vi "Data Parameters FG.vi"(7 "Action":T1, 8 "error in (no error)":errorcluster, 10 "Data Parameters":T3={"Data Type"=enum."Single Channel", "Channel Type"=enum."Format", "Format String"="%.3g", "Expected String"="", "Type"=enum."SGL", "List"=[], "Delimiter"=","}, 11 "Item Ref in":T2 format="%.0x") -> (0 "error out":errorcluster, 2 "Data Parameters":T3={"Data Type"=enum."Single Channel", "Channel Type"=enum."Format", "Format String"="%.3g", "Expected String"="", "Type"=enum."SGL", "List"=[], "Delimiter"=","}, 3 "Item Ref out":T2 format="%.0x")   [LabVIEW 2015, in "Instrument Addon Shared.lvlib"]
uses:
  Instrument Addon Shared.lvlib
  Types/Data Parameters.ctl
  Types/Protocol Data Type.ctl
  Types/Data Channel Type.ctl
  Types/Type Cast Type.ctl
  <vilib>/NI Veristand/Custom Device API/Custom Device Item Ref.ctl
  Types/FG Control.ctl
  <vilib>/NI Veristand/Custom Device API/Set Item Property (String).vi
  <vilib>/NI Veristand/Custom Device API/Set Item Property (String Array).vi
  <vilib>/NI Veristand/Custom Device API/Set Item Property (U32).vi
  <vilib>/NI Veristand/Custom Device API/Get Item Property (String).vi
  <vilib>/NI Veristand/Custom Device API/Get Item Property (String Array).vi
  <vilib>/NI Veristand/Custom Device API/Get Item Property (U32).vi
  Constants.vi
  <vilib>/NI VeriStand/Custom Device API/Custom Device API.lvlib
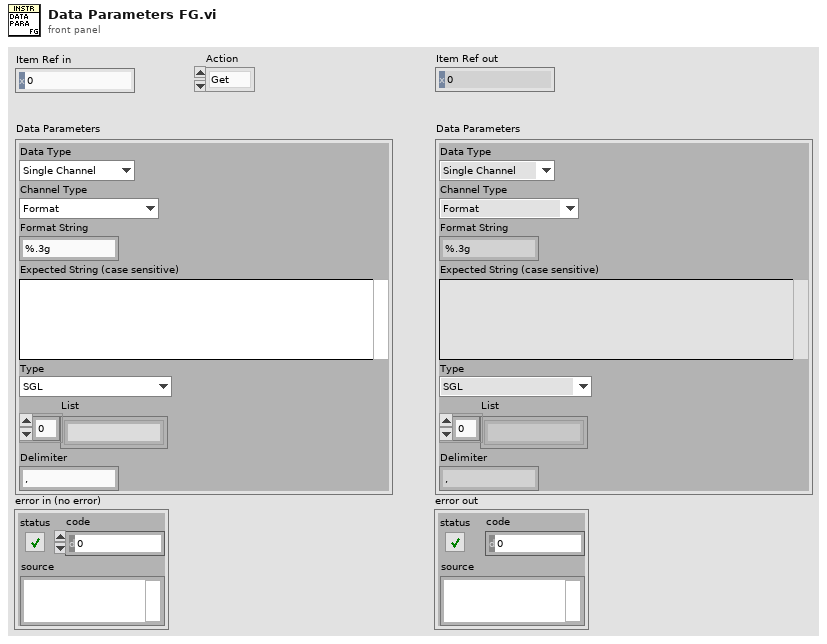
[diagram p1: front panel]
types:
  T1 = typedef "Instrument Addon Shared.lvlib/FG Control.ctl" = enum16{"Get", "Set"}
  T2 = typedef "Custom Device API.lvlib/Custom Device Item Ref.ctl" = u64
  T3 = typedef "Instrument Addon Shared.lvlib/Data Parameters.ctl" = cluster{"Data Type":T4, "Channel Type":T5, "Format String":string, "Expected String":string, "Type":T6, "List":string[], "Delimiter":string}
  T4 = typedef "Instrument Addon Shared.lvlib/Protocol Data Type.ctl" = enum16{"Single Channel", "Array"}
  T5 = typedef "Instrument Addon Shared.lvlib/Data Channel Type.ctl" = enum16{"Format", "Comparison", "Type Cast", "Enumerated List"}
  T6 = typedef "Instrument Addon Shared.lvlib/Type Cast Type.ctl" = enum16{"DBL", "SGL", "U64", "U32", "U16", "U8", "I64", "I32", "I16", "I8"}
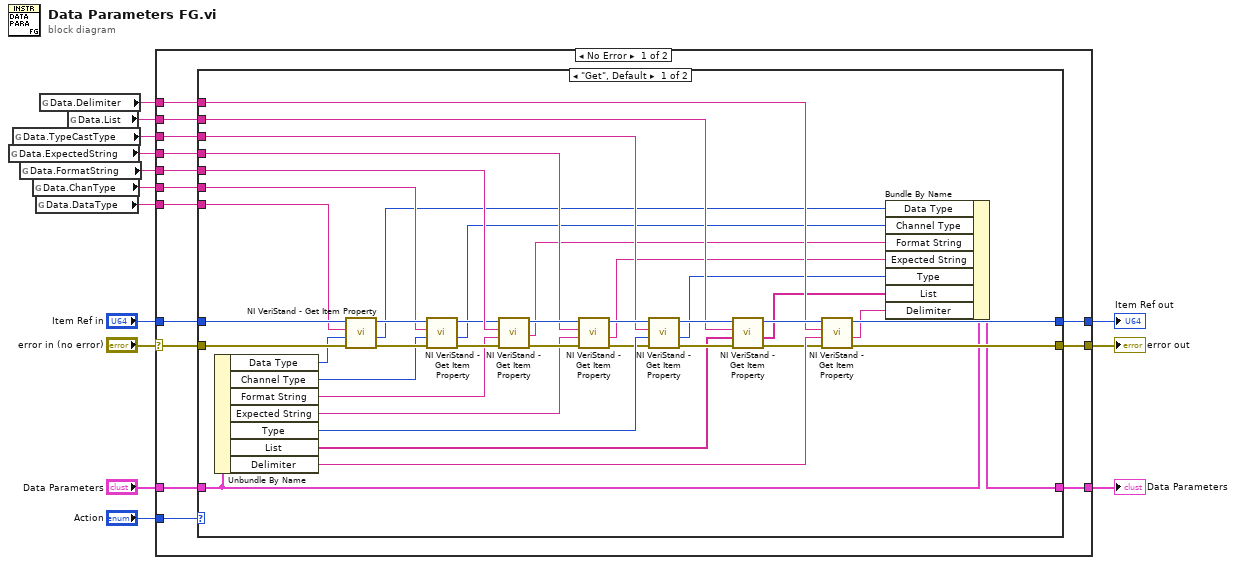
[diagram p0: block diagram]
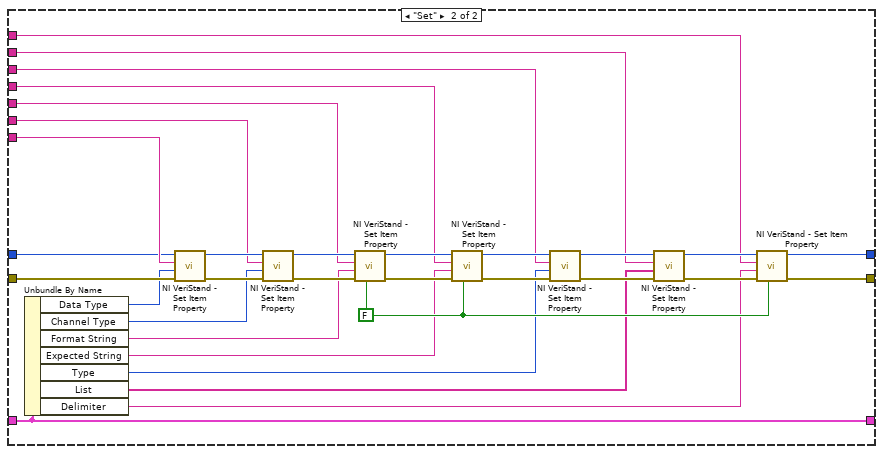
[diagram p2: hidden frame]
diagram:
  n1 = global read "Constants.vi" "Data.ExpectedString"() -> (w4:string)
  n2 = global read "Constants.vi" "Data.TypeCastType"() -> (w3:string)
  n3 = global read "Constants.vi" "Data.FormatString"() -> (w5:string)
  n4 = global read "Constants.vi" "Data.ChanType"() -> (w6:string)
  n5 = global read "Constants.vi" "Data.DataType"() -> (w8:string)
  n6 = global read "Constants.vi" "Data.Delimiter"() -> (w1:string)
  n7 = global read "Constants.vi" "Data.List"() -> (w2:string)
  n8 = case shown="No Error" "error in (no error)" {
    selector: "error in (no error)" -> [w23 w102]
    tunnel: w8 -> [w28 _]
    tunnel: [w27 w100] -> w12
    tunnel: "Item Ref in" -> [w26 w100]
    tunnel: "Data Parameters" -> [w25 w101]
    tunnel: [w24 w102] -> w11
    tunnel: [w22 w101] -> w7
    tunnel: "Action" -> [w21 _]
    tunnel: w6 -> [w20 _]
    tunnel: w5 -> [w19 _]
    tunnel: w4 -> [w18 _]
    tunnel: w3 -> [w17 _]
    tunnel: w2 -> [w16 _]
    tunnel: w1 -> [w15 _]
    frame No Error {
      n9 = case shown="\"Get\", Default" w21 {
        tunnel: w28 -> [w65 w99]
        tunnel: [w42 w82] -> w27
        tunnel: w26 -> [w66 w98]
        tunnel: w25 -> [w37 w96]
        tunnel: [w46 w83] -> w24
        tunnel: w23 -> [w67 w97]
        tunnel: [w36 w96] -> w22
        tunnel: w20 -> [w60 w73]
        tunnel: w19 -> [w59 w72]
        tunnel: w18 -> [w41 w71]
        tunnel: w17 -> [w40 w70]
        tunnel: w16 -> [w39 w69]
        tunnel: w15 -> [w38 w68]
        frame "Get", Default {
          n10 = Unbundle By Name(w37) -> ("Data Type"=w64:T4, "Channel Type"=w61:T5, "Format String"=w56:string, "Expected String"=w53:string, "Type"=w52:T6, "List"=w48:string[], "Delimiter"=w47:string)
          n11 = call-poly <vilib>:"NI VeriStand - Get Item Property.vi"("error in (no error)"=w67, "Default Value"=w64, "Property Name"=w65, "Item Ref in"=w66) -> ("error out"=w62:errorcluster, "Value"=w29:u32, "Item Ref out"=w63:T2)  [unwired: 4 in, 1 out]
          n12 = call-poly <vilib>:"NI VeriStand - Get Item Property.vi"("error in (no error)"=w62, "Default Value"=w61, "Property Name"=w60, "Item Ref in"=w63) -> ("error out"=w57:errorcluster, "Value"=w30:u32, "Item Ref out"=w58:T2)  [unwired: 4 in, 1 out]
          n13 = call-poly <vilib>:"NI VeriStand - Get Item Property.vi"("error in (no error)"=w57, "Default Value"=w56, "Property Name"=w59, "Item Ref in"=w58) -> ("error out"=w54:errorcluster, "Value"=w31:string, "Item Ref out"=w55:T2)  [unwired: 4 in, 1 out]
          n14 = call-poly <vilib>:"NI VeriStand - Get Item Property.vi"("error in (no error)"=w54, "Default Value"=w53, "Property Name"=w41, "Item Ref in"=w55) -> ("error out"=w51:errorcluster, "Value"=w32:string, "Item Ref out"=w50:T2)  [unwired: 4 in, 1 out]
          n15 = call-poly <vilib>:"NI VeriStand - Get Item Property.vi"("error in (no error)"=w51, "Default Value"=w52, "Property Name"=w40, "Item Ref in"=w50) -> ("error out"=w49:errorcluster, "Value"=w33:u32, "Item Ref out"=w44:T2)  [unwired: 4 in, 1 out]
          n16 = call-poly <vilib>:"NI VeriStand - Get Item Property.vi"("error in (no error)"=w49, "Default Value"=w48, "Property Name"=w39, "Item Ref in"=w44) -> ("error out"=w45:errorcluster, "Value"=w34:string[], "Item Ref out"=w43:T2)  [unwired: 4 in, 1 out]
          n17 = call-poly <vilib>:"NI VeriStand - Get Item Property.vi"("error in (no error)"=w45, "Default Value"=w47, "Property Name"=w38, "Item Ref in"=w43) -> ("error out"=w46:errorcluster, "Value"=w35:string, "Item Ref out"=w42:T2)  [unwired: 4 in, 1 out]
          n18 = Bundle By Name(cluster=w37, "Data Type"=w29, "Channel Type"=w30, "Format String"=w31, "Expected String"=w32, "Type"=w33, "List"=w34, "Delimiter"=w35) -> (w36:T3)
        }
        frame "Set" {
          w78 = FALSE ("Binary String (T)")
          n19 = Unbundle By Name(w96) -> ("Data Type"=w81:T4, "Channel Type"=w80:T5, "Format String"=w79:string, "Expected String"=w77:string, "Type"=w76:T6, "List"=w75:string[], "Delimiter"=w74:string)
          n20 = call-poly <vilib>:"NI VeriStand - Set Item Property.vi"("error in (no error)"=w97, "Value"=w81, "Property Name"=w99, "Item Ref in"=w98) -> ("error out"=w94:errorcluster, "Item Ref out"=w95:T2)  [unwired: 5 in, 1 out]
          n21 = call-poly <vilib>:"NI VeriStand - Set Item Property.vi"("error in (no error)"=w94, "Value"=w80, "Property Name"=w73, "Item Ref in"=w95) -> ("error out"=w92:errorcluster, "Item Ref out"=w93:T2)  [unwired: 5 in, 1 out]
          n22 = call-poly <vilib>:"NI VeriStand - Set Item Property.vi"("Binary String (T)"=w78, "error in (no error)"=w92, "Value"=w79, "Property Name"=w72, "Item Ref in"=w93) -> ("error out"=w90:errorcluster, "Item Ref out"=w91:T2)  [unwired: 4 in, 1 out]
          n23 = call-poly <vilib>:"NI VeriStand - Set Item Property.vi"("Binary String (T)"=w78, "error in (no error)"=w90, "Value"=w77, "Property Name"=w71, "Item Ref in"=w91) -> ("error out"=w88:errorcluster, "Item Ref out"=w89:T2)  [unwired: 4 in, 1 out]
          n24 = call-poly <vilib>:"NI VeriStand - Set Item Property.vi"("error in (no error)"=w88, "Value"=w76, "Property Name"=w70, "Item Ref in"=w89) -> ("error out"=w87:errorcluster, "Item Ref out"=w86:T2)  [unwired: 5 in, 1 out]
          n25 = call-poly <vilib>:"NI VeriStand - Set Item Property.vi"("error in (no error)"=w87, "Value"=w75, "Property Name"=w69, "Item Ref in"=w86) -> ("error out"=w85:errorcluster, "Item Ref out"=w84:T2)  [unwired: 5 in, 1 out]
          n26 = call-poly <vilib>:"NI VeriStand - Set Item Property.vi"("Binary String (T)"=w78, "error in (no error)"=w85, "Value"=w74, "Property Name"=w68, "Item Ref in"=w84) -> ("error out"=w83:errorcluster, "Item Ref out"=w82:T2)  [unwired: 4 in, 1 out]
        }
      }
    }
    frame Error {
    }
  }
  "error out" <- w11
  "Data Parameters" <- w7
  "Item Ref out" <- w12
